vi "Close and Open a Relay.vi"(0 "Relays to Toggle":T1, 5 "Settling Time(s)":dbl, 11 "error in":errorcluster) -> (15 "error out":errorcluster)   [LabVIEW 2019]
uses:
  SubVIs/TSM SSC Relay.ctl
  <vilib>/NI_TestStand_SemiconductorModule/NI_TestStand_Semiconductor_Module.lvlibp/PinMap/PinQueryContext/MultiplePinMultipleSessionQueryContext/MultiplePinMultipleSessionQueryContext.lvclass
  <vilib>/NI_TestStand_SemiconductorModule/NI_TestStand_Semiconductor_Module.lvlibp/PinMap/General/SemiconductorModuleContext.ctl
  SSC/SSC Relay.ctl
  SubVIs/TSM Filtered Pins Info.ctl
  <instrlib>/niSwitch/niSwitch.llb/niSwitch Relay Action.ctl
  SSC/SSC Relay Control.vi
  SSC/SSC Relay Control/SSC Relay Control Single Action.vi
  SSC/SSC Relay Control Core.vi
  SSC/Single SSC Relay NI-Switch Control.vi
  SSC/Single SSC Relay Fill Additional Error info.vi
  SSC/SSC Relay Expand Action Array to All Sessions.vi
  <vilib>/Utility/error.llb/Error Cluster From Error Code.vi
  <instrlib>/niSwitch/niSwitch.llb/niSwitch Get Relay Position.vi
  <instrlib>/niSwitch/niSwitch.llb/niSwitch Relay Control.vi
  <vilib>/Utility/High Resolution Polling Wait.vi
  <vilib>/NI_TestStand_SemiconductorModule/NI_TestStand_Semiconductor_Module.lvlibp
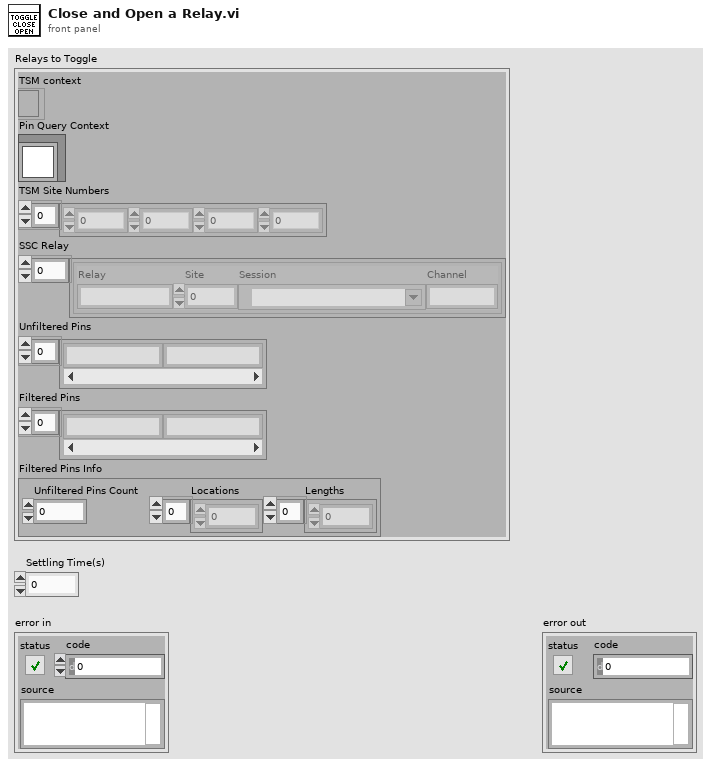
[diagram p1: front panel]
types:
  T1 = typedef "TSM SSC Relay.ctl" = cluster{"TSM context":T2, "Pin Query Context":refnum<class "MultiplePinMultipleSessionQueryContext.lvclass">, "TSM Site Numbers":i32[], "SSC Relay":T3[], "Unfiltered Pins":string[], "Filtered Pins":string[], "Filtered Pins Info":T4}
  T2 = typedef "NI_TestStand_Semiconductor_Module.lvlibp/SemiconductorModuleContext.ctl" = refnum<k7>
  T3 = typedef "SSC Relay.ctl" = cluster{"Relay":string, "Site":i32, "Session":refnum<k15>, "Channel":string}
  T4 = typedef "TSM Filtered Pins Info.ctl" = cluster{"Unfiltered Pins Count":i32, "Locations":i32[], "Lengths":i32[]}
  T5 = typedef "niSwitch Relay Action.ctl" = i32
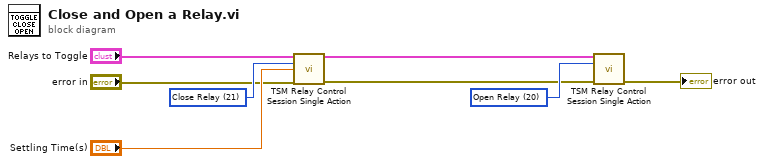
[diagram p0: block diagram]
diagram:
  w7 = T5 21 items=["Open Relay"=20, "Close Relay"=21] ("Relay Action")
  w5 = T5 20 items=["Open Relay"=20, "Close Relay"=21] ("Relay Action")
  n1 = call "TSM Relay Control Session Single Action.vi"("TSM Relay in"="Relays to Toggle", "Relay Action"=w7, "Settling Time (s)"="Settling Time(s)", "error in"="error in") -> ("TSM Relay out"=w1:T1, "error out"=w4:errorcluster)  [unwired: 9 in, 1 out]
  n2 = call "TSM Relay Control Session Single Action.vi"("TSM Relay in"=w1, "Relay Action"=w5, "error in"=w4) -> ("error out"=→"error out":errorcluster)  [unwired: 10 in, 2 out]
